vi "SigProc_subVI Mmode.vi"(1 "Y Data":dbl[](array[numeric])) -> (0 "element":dbl)   [LabVIEW 2018, in "Sig2MS.lvclass"]
uses:
  Sig2MS.lvclass
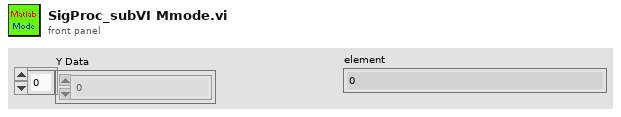
[diagram p1: front panel]
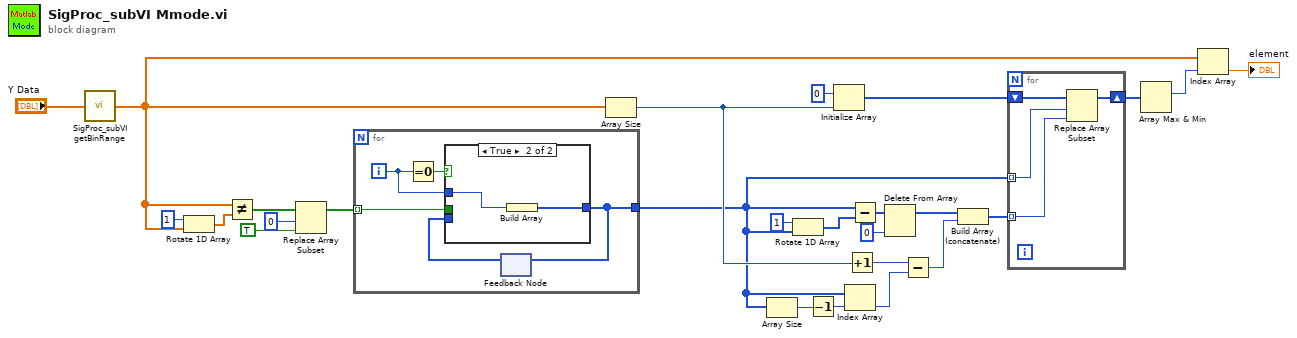
[diagram p0: block diagram]
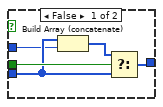
[diagram p2: hidden frame]
diagram:
  n1 = call "SigProc_subVI getBinRange.vi"("Y Data"="Y Data") -> ("Valid Data"=w1:dbl[])
  n2 = Rotate 1D Array(1:w1, 2:1 ("n")) -> (0:w24:dbl[])
  n3 = Not Equal?(x=w1, y=w24) -> (x != y?=w23:bool[])
  n4 = Replace Array Subset(array=w23, new element=TRUE ("new element/subarray"), index=0) -> (w19:bool[])
  n5 = for {
    tunnel: w19 -> [w31] mode=indexing
    tunnel: [w27] -> w3
    i -> [w29]
    n6 = Equal To 0?(x=w29) -> (x = 0?=w30:bool)
    n7 = feedback #1() -> (w28:i32[])  [unwired: 1 in]
    n8 = case shown="True" w30 {
      tunnel: w31 -> [w36 _]
      tunnel: w29 -> [w34 w38]
      tunnel: [w32 w37] -> w27
      tunnel: w28 -> [w35 _]
      frame False {
        n9 = Build Array (concatenate)(w35, w34) -> (w33:i32[])
        n10 = Select(t=w33, s=w36, f=w35) -> (s? t:f=w32:i32[])
      }
      frame True {
        n11 = Build Array(w38) -> (w37:i32[])
      }
    }
    n12 = feedback-in #1(w27) -> ()
  }
  n13 = Array Size(array=w1) -> (size(s)=w12:i32)
  n14 = Array Size(array=w3) -> (size(s)=w15:i32)
  n15 = Rotate 1D Array(1:w3, 2:1 ("n")) -> (0:w2:i32[])
  n16 = Decrement(x=w15) -> (x-1=w14:i32)
  n17 = Initialize Array(0 ("element"), w12) -> (w13:i32[])
  n18 = Index Array(array=w3, index=w14) -> (element=w10:i32)
  n19 = Increment(x=w12) -> (x+1=w11:i32)
  n20 = Subtract(x=w3, y=w2) -> (x-y=w17:i32[])
  n21 = Delete From Array(array=w17, index=0) -> (array with subset deleted=w9:i32[])  [unwired: 1 in, 1 out]
  n22 = Subtract(x=w11, y=w10) -> (x-y=w8:i32)
  n23 = Build Array (concatenate)(w9, w8) -> (w7:i32[])
  n24 = for {
    tunnel: w7 -> [w40] mode=indexing
    tunnel: w3 -> [w41] mode=indexing
    shift-right: [w39] -> w6
    shift-left: w13 -> [w42]
    n25 = Replace Array Subset(array=w42, new element=w40, index=w41) -> (w39:i32[])
  }
  n26 = Array Max & Min(array=w6) -> (max index (indices)=w5:i32)  [unwired: 3 out]
  n27 = Index Array(array=w1, index=w5) -> (element=→"element":dbl)
